vi "scanDeviceGlobalVarsWrite.vi"(0 "ChooseScanDevice":bool, 8 "internalDacAvailable":bool, 11 "ScanDevice":enum16{"internal DAC", "external Python"}(ring)) -> ()   [LabVIEW 2014]
uses:
  <vilib>/rvi/Emulation/niFpgaSctlEmulationGetInTimedLoop.vi
  scanDeviceGlobalVars.vi
  <vilib>/rvi/Emulation/niFpgaProcessEmulError.vi
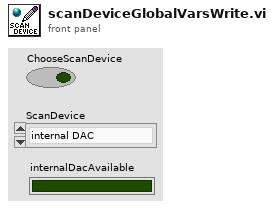
[diagram p1: front panel]
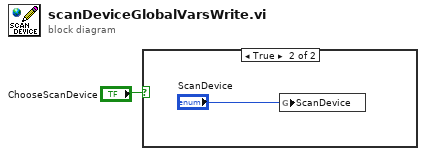
[diagram p0: block diagram]
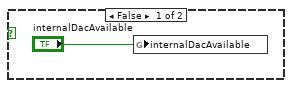
[diagram p2: hidden frame]
diagram:
  n1 = case shown="True" "ChooseScanDevice" {
    frame False {
      n2 = global write "scanDeviceGlobalVars.vi" "internalDacAvailable"("internalDacAvailable") -> ()
    }
    frame True {
      n3 = global write "scanDeviceGlobalVars.vi" "ScanDevice"("ScanDevice") -> ()
    }
  }
